vi "Load Settings.vi"(8 "error in (no error)":errorcluster, 11 "Settings in":refnum<class "Settings.lvclass">) -> (0 "error out":errorcluster, 3 "Settings out":refnum<class "Settings.lvclass">)   [LabVIEW 2010, in "Settings.lvclass"]
uses:
  Settings.lvclass
  Settings.lvclass/Settings.ctl
  <vilib>/Utility/xml.llb/Read From XML File(string).vi
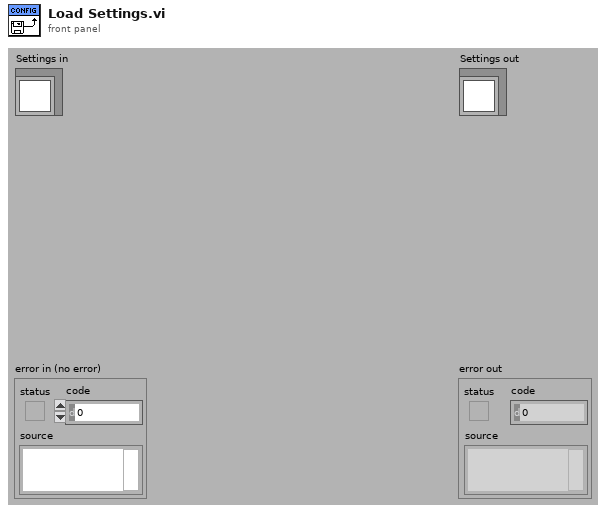
[diagram p1: front panel]
types:
  T1 = cluster{"Dye Name":string, "Pulse Sequence":cluster{"LED Name":string, "Pulse Length (s)":dbl, "Delay Before (s)":dbl, "Delay After (s)":dbl, "Trigger Camera":bool}[], "Emission Filter":i16, "Exposure (s)":dbl, "Yellow Select":bool, "# Pulses":i32}[]
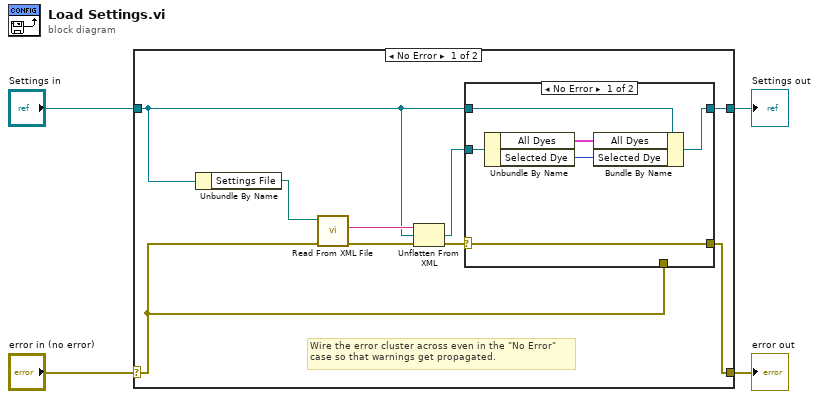
[diagram p0: block diagram]
diagram:
  n1 = case shown="No Error" "error in (no error)" {
    selector: "error in (no error)" -> [w5 w23]
    tunnel: [w6 w23] -> w3
    tunnel: [w8 w22] -> w1
    tunnel: "Settings in" -> [w9 w22]
    frame No Error {
      # "Wire the error cluster across even in the \"No Error\"\ncase so that warnings get propagated."
      n2 = Unbundle By Name(w9) -> ("Settings File"=w11:path)
      n3 = call-poly <vilib>:"Read From XML File.vi"("error in (no error)"=w5, "XML File Path"=w11) -> ("error out"=w12:errorcluster, "XML Elements"=w13:string)  [unwired: 7 in, 1 out]
      n4 = Unflatten From XML(xml string=w13, type=w9, error in (no error)=w12) -> (value=w10:refnum<class "Settings.lvclass">, error out=w7:errorcluster)
      n5 = case shown="No Error" w7 {
        selector: w7 -> [w14 _]
        tunnel: w10 -> [w19 _]
        tunnel: w9 -> [w18 w21]
        tunnel: [w17 w21] -> w8
        tunnel: [w14 w20] -> w6
        tunnel: w5 -> [_ w20]
        frame No Error {
          n6 = Unbundle By Name(w19) -> ("All Dyes"=w16:T1, "Selected Dye"=w15:i32)
          n7 = Bundle By Name(cluster=w18, "All Dyes"=w16, "Selected Dye"=w15) -> (w17:refnum<class "Settings.lvclass">)
        }
        frame Error {
        }
      }
    }
    frame Error {
    }
  }
  "error out" <- w3
  "Settings out" <- w1
